vi "CamWatcher.vi"(11 "Rotation Count":dbl) -> (3 "Rotation Count":dbl)   [LabVIEW 2012]
uses:
  Autonomous_Routine_Global.vi
panel:
  out "x+y":dbl
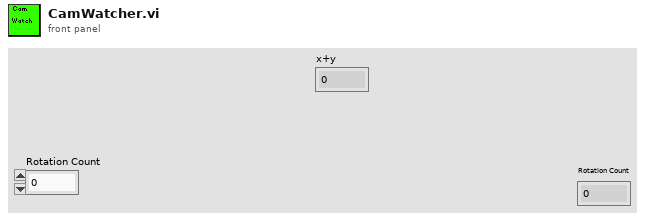
[diagram p1: front panel]
types:
  T1 = typedef "WPI_AnalogChannelDevRef.ctl" = cluster{"DevStatus":errorcluster, "Analog Module":T2, "Analog Channel":T3}
  T2 = typedef "FPGA_TypedefAnalogModule.ctl" = enum16{"Analog Module 1", "Analog Module 2"}
  T3 = typedef "FPGA_AIChannel.ctl" = enum8{"AI 1", "AI 2", "AI 3", "AI 4", "AI 5", "AI 6", "AI 7", "AI 8", "Invalid"}
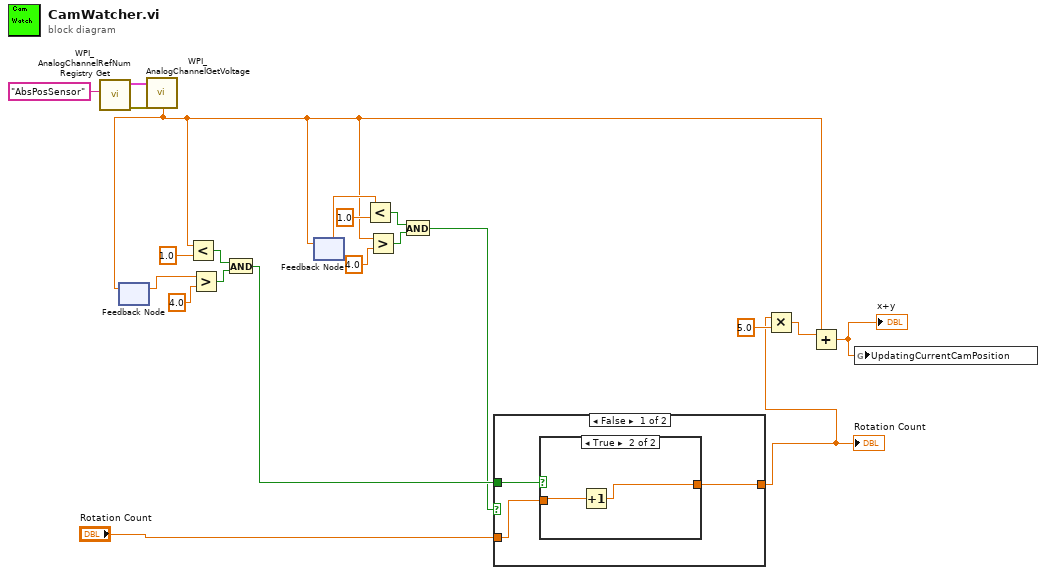
[diagram p0: block diagram]
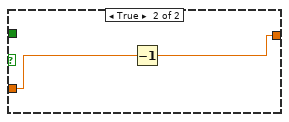
[diagram p3: hidden frame]
diagram:
  n1 = call <vilib>:"WPI_AnalogChannelRefNum Registry Get.vi"("refnum name"="AbsPosSensor") -> ("error out"=w21:errorcluster, "AIDeviceRef"=w20:T1)  [unwired: 9 in]
  n2 = feedback #1() -> (w2:dbl)  [unwired: 1 in]
  n3 = call <vilib>:"WPI_AnalogChannelGetVoltage.vi"("error in (no error)"=w21, "AIDeviceRef"=w20) -> ("Voltage"=w1:dbl)  [unwired: 7 in, 2 out]
  n4 = feedback-in #1(w1) -> ()
  n5 = Less?(x=w1, y=1.0) -> (x < y?=w11:bool)
  n6 = Greater?(x=w2, y=4.0) -> (0:w10:bool)
  n7 = And(x=w11, y=w10) -> (x .and. y?=w5:bool)
  n8 = feedback #2() -> (w3:dbl)  [unwired: 1 in]
  n9 = feedback-in #2(w1) -> ()
  n10 = Less?(x=w3, y=1.0) -> (x < y?=w8:bool)
  n11 = Greater?(x=w1, y=4.0) -> (0:w9:bool)
  n12 = And(x=w8, y=w9) -> (x .and. y?=w4:bool)
  n13 = case shown="False" w4 {
    tunnel: "Rotation Count" -> [w24 w28]
    tunnel: [w23 w29] -> w14
    tunnel: w5 -> [w22 _]
    frame False {
      n14 = case shown="True" w22 {
        tunnel: w24 -> [w25 w27]
        tunnel: [w25 w26] -> w23
        frame False {
        }
        frame True {
          n15 = Increment(x=w27) -> (x+1=w26:dbl)
        }
      }
    }
    frame True {
      n16 = Decrement(x=w28) -> (x-1=w29:dbl)
    }
  }
  "Rotation Count" <- w14
  n17 = Multiply(x=w14, y=5.0) -> (x*y=w16:dbl)
  n18 = Add(x=w16, y=w1) -> (x+y=w17:dbl)
  "x+y" <- w17
  n19 = global write "Autonomous_Routine_Global.vi" "UpdatingCurrentCamPosition"(w17) -> ()
